vi "Read_DID.vi"() -> ()   [LabVIEW 2014]
uses:
  housekeeper/MSI/MSI typedefs/MSI.ctl
  <vilib>/Utility/error.llb/DialogType.ctl
panel:
  out "instant datarun":T1
  out "time stamp":timestamp
  in  "stop instantaneous loop":bool
  out "Shot collection loop":i32
  out "North discharge voltage":sgl[](graph)
  out "NDV error":errorcluster
  out "North discharge current":sgl[](graph)
  out "NDC error":errorcluster
  out "Shots in queue":i32
  out "Data request error":errorcluster
  in  "stop TCP listen":bool
  in  "Num diodes":i32=3
  in  "Num interferometers":i32=1
  out "Shot send loop":i32
  out "MSI+DID string length":i32
  out "TCP error":errorcluster
  out "Queue overflowed":bool
  in  "stop TCP":bool
  in  "stop DID":bool
  out "Data run status":T2 {"Timestamp" format="%#_8g"}
  out "MSI timed out":bool
  out "MSI error":errorcluster
  out "MSI":T3={"Timestamp"=0.0, "Discharge"={"Data valid"=FALSE, "Discharge current"=[], "Cathode anode voltage"=[], "Pulse length"=0.0, "Peak current"=0.0, "Bank voltage"=0.0}, "Heater"={"Data valid"=FALSE, "Heater current"=0.0, "Heater voltage"=0.0, "Heater temperature"=0.0}, "Gas pressure"={"Ion gauge data valid"=FALSE, "RGA data valid"=FALSE, "Fill pressure"=0.0, "Peak AMU"=0.0, "RGA partial pressures"=[]}, "Magnetic field"={"Data valid"=FALSE, "Magnetic field profile"=[], "Magnet power supply currents"=[], "Peak magnetic field"=0.0}, "Interferometer array"=[{"Data valid"=TRUE, "Interferometer"=[1200000000000.0, 1300000000000.0, 1500000000000.0, 1400000000000.0], "Peak density"=347.7}, {"Data valid"=TRUE, "Interferometer"=[1330000000000.0, 1450000000000.0, 1430000000000.0, 1560000000000.0], "Peak density"=654.9}, {"Data valid"=TRUE, "Interferometer"=[1110000000000.0, 1130000000000.0, 1440000000000.0, 1250000000000.0], "Peak density"=45.0}]} {"Timestamp" format="%<%X\n%x>T"}
  out "No discharge":bool
  in  "Write DID to file?":bool=TRUE
  out "File error":errorcluster
  out "Run error":errorcluster
  out "DID+MSI string":string
  out "Save path":path
  out "Data run timed out":bool
  out "Diode array":dbl[][](graph)
  out "Diode array":waveform(dbl)[](array[waveform])
  out "Diode error":errorcluster
  out "Micorwave array":dbl[][](graph)
  out "Microwave array":waveform(dbl)[](array[waveform])
  out "MArray error":errorcluster
  out "Discharge voltage":sgl[](graph)
  out "DV error":errorcluster
  out "Discharge current":sgl[](graph)
  out "DC error":errorcluster
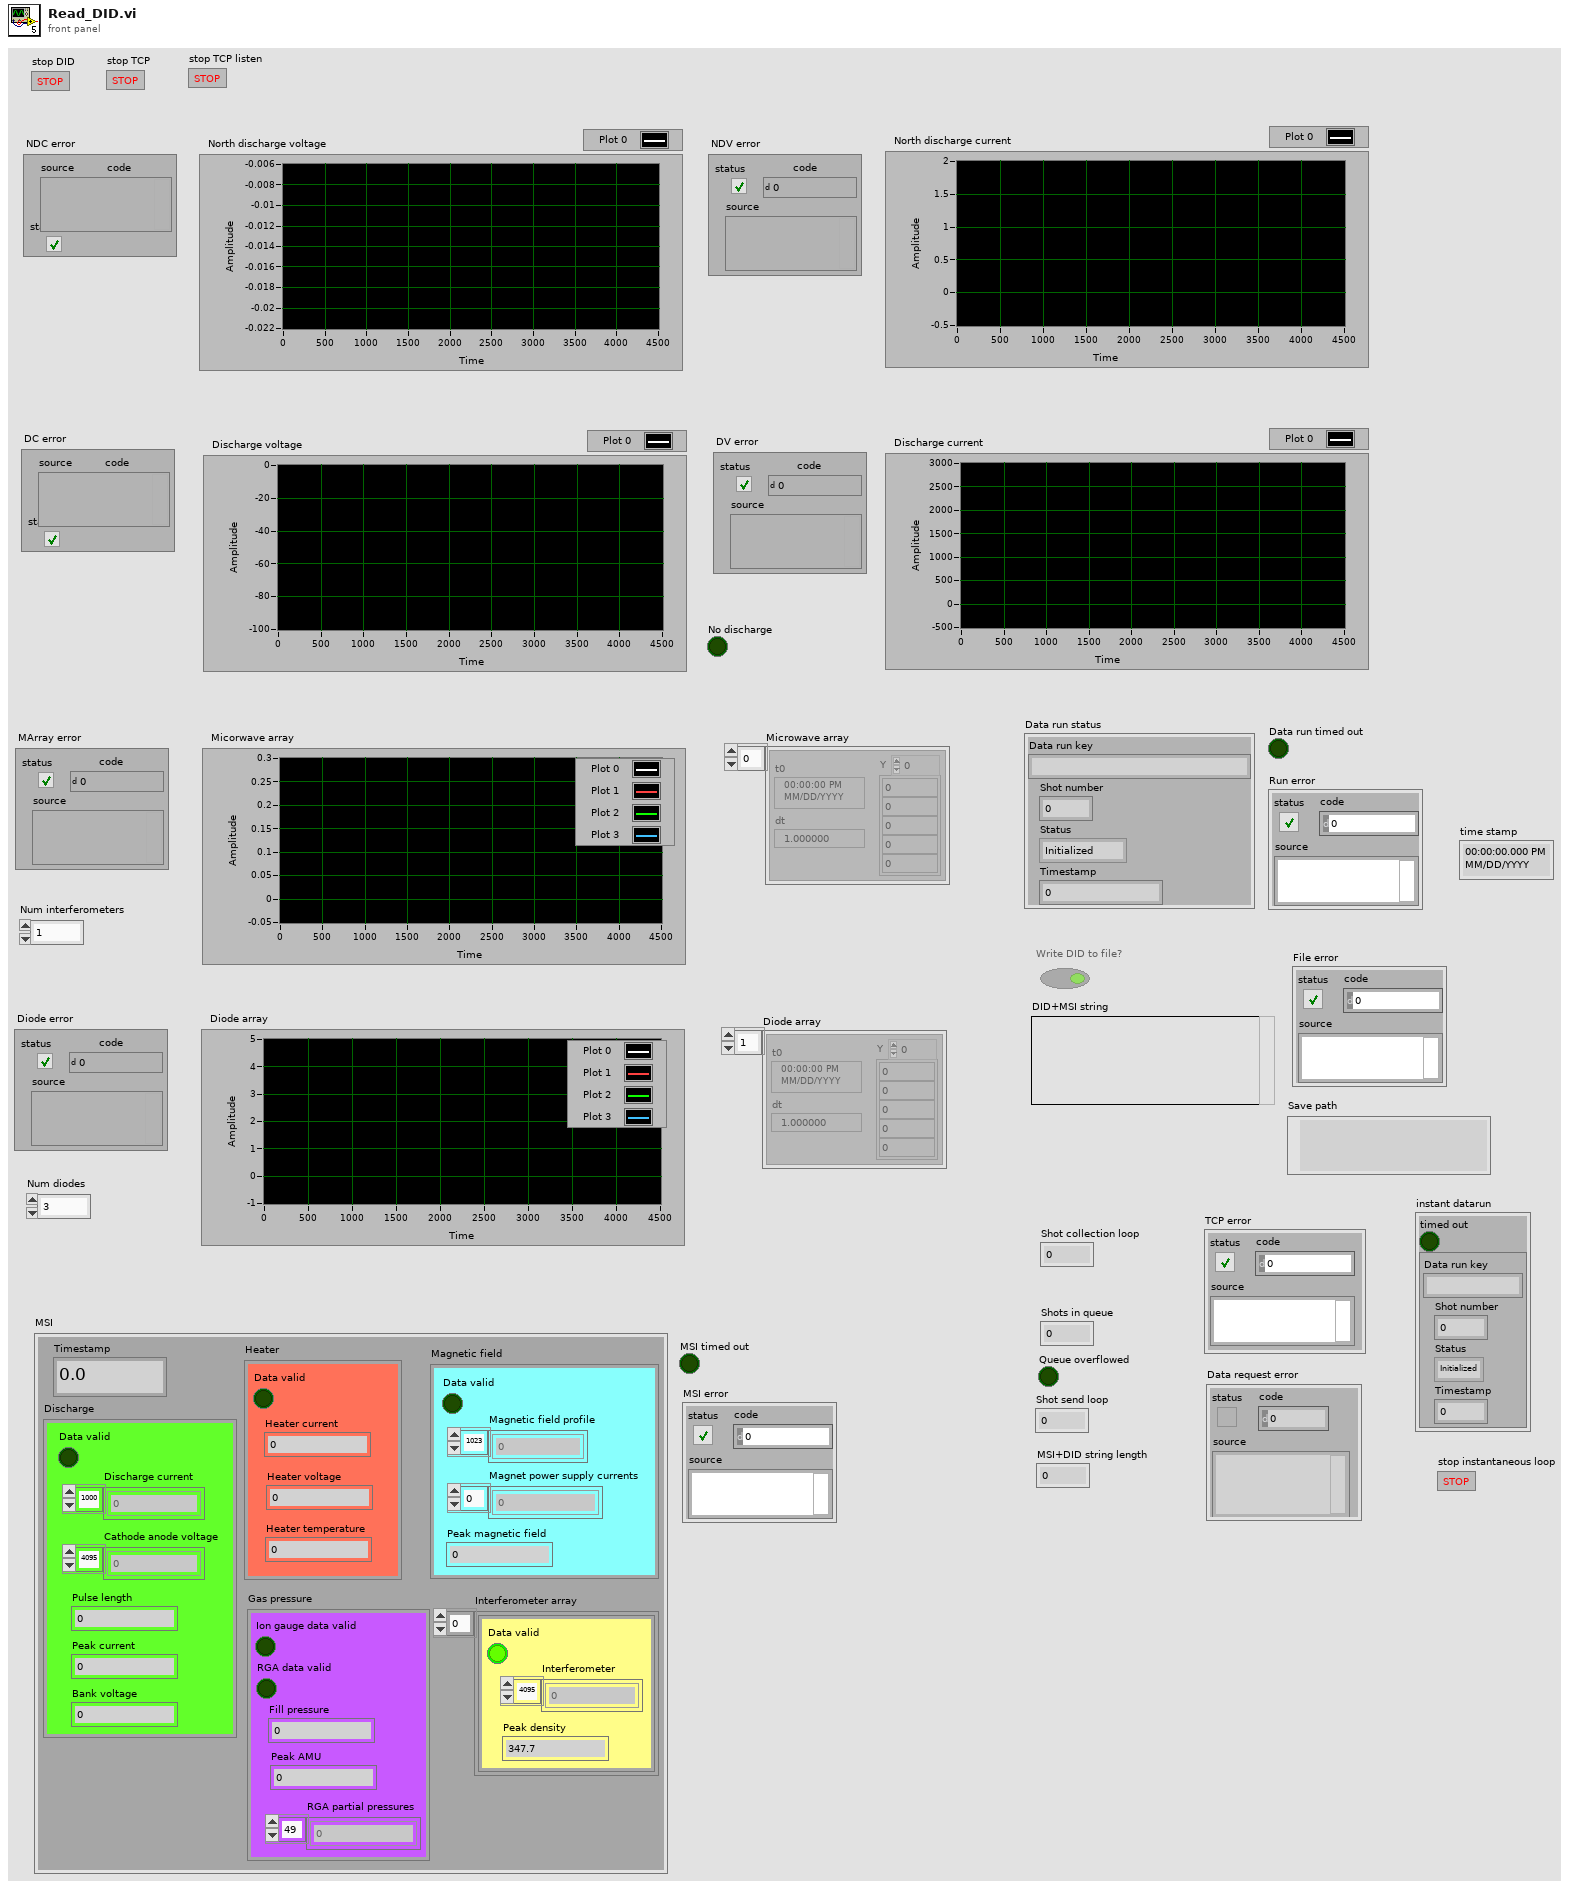
[diagram p1: front panel]
types:
  T1 = cluster{"timed out":bool, cluster{"Data run key":string, "Shot number":u32, "Status":enum16{"Initialized", "Running", "Aborted", "Default"}, "Timestamp":dbl}}
  T2 = cluster{"Data run key":string, "Shot number":u32, "Status":enum16{"Initialized", "Running", "Aborted", "Default"}, "Timestamp":dbl}
  T3 = typedef "MSI.ctl" = cluster{"Timestamp":dbl, "Discharge":cluster{"Data valid":bool, "Discharge current":sgl[], "Cathode anode voltage":sgl[], "Pulse length":sgl, "Peak current":sgl, "Bank voltage":sgl}, "Heater":cluster{"Data valid":bool, "Heater current":sgl, "Heater voltage":sgl, "Heater temperature":sgl}, "Gas pressure":cluster{"Ion gauge data valid":bool, "RGA data valid":bool, "Fill pressure":sgl, "Peak AMU":sgl, "RGA partial pressures":sgl[]}, "Magnetic field":cluster{"Data valid":bool, "Magnetic field profile":sgl[], "Magnet power supply currents":sgl[], "Peak magnetic field":sgl}, "Interferometer array":cluster{"Data valid":bool, "Interferometer":sgl[], "Peak density":sgl}[]}
  T4 = enum16{"Initialized", "Running", "Aborted", "Default"}
  T5 = enum16{"open", "replace", "create", "open or create", "replace or create", "replace or create with confirmation"}
  T6 = cluster{bool, cluster{"Data run key":string, "Shot number":u32, "Status":enum16{"Initialized", "Running", "Aborted", "Default"}, "Timestamp":dbl}}
  T7 = typedef "DialogType.ctl" = u16
  T8 = cluster{"Data valid":bool, "Heater current":sgl, "Heater voltage":sgl, "Heater temperature":sgl}
  T9 = cluster{"Ion gauge data valid":bool, "RGA data valid":bool, "Fill pressure":sgl, "Peak AMU":sgl, "RGA partial pressures":sgl[]}
  T10 = cluster{"Data valid":bool, "Magnetic field profile":sgl[], "Magnet power supply currents":sgl[], "Peak magnetic field":sgl}
  T11 = cluster{"timed out":bool, "Timestamp":dbl, "Heater":cluster{"Data valid":bool, "Heater current":sgl, "Heater voltage":sgl, "Heater temperature":sgl}, "Gas pressure":cluster{"Ion gauge data valid":bool, "RGA data valid":bool, "Fill pressure":sgl, "Peak AMU":sgl, "RGA partial pressures":sgl[]}, "Magnetic field":cluster{"Data valid":bool, "Magnetic field profile":sgl[], "Magnet power supply currents":sgl[], "Peak magnetic field":sgl}}
  T12 = cluster{"Waveform Graph 4":sgl[], "Waveform Graph 4":sgl[], "Waveform Graph 4":sgl[], "Waveform Graph 4":sgl[], "Y":dbl[][], timestamp[], dbl[], "Y":dbl[][], timestamp[], dbl[], "timed out":bool, cluster{"Data run key":string, "Shot number":u32, "Status":enum16{"Initialized", "Running", "Aborted", "Default"}, "Timestamp":dbl}}
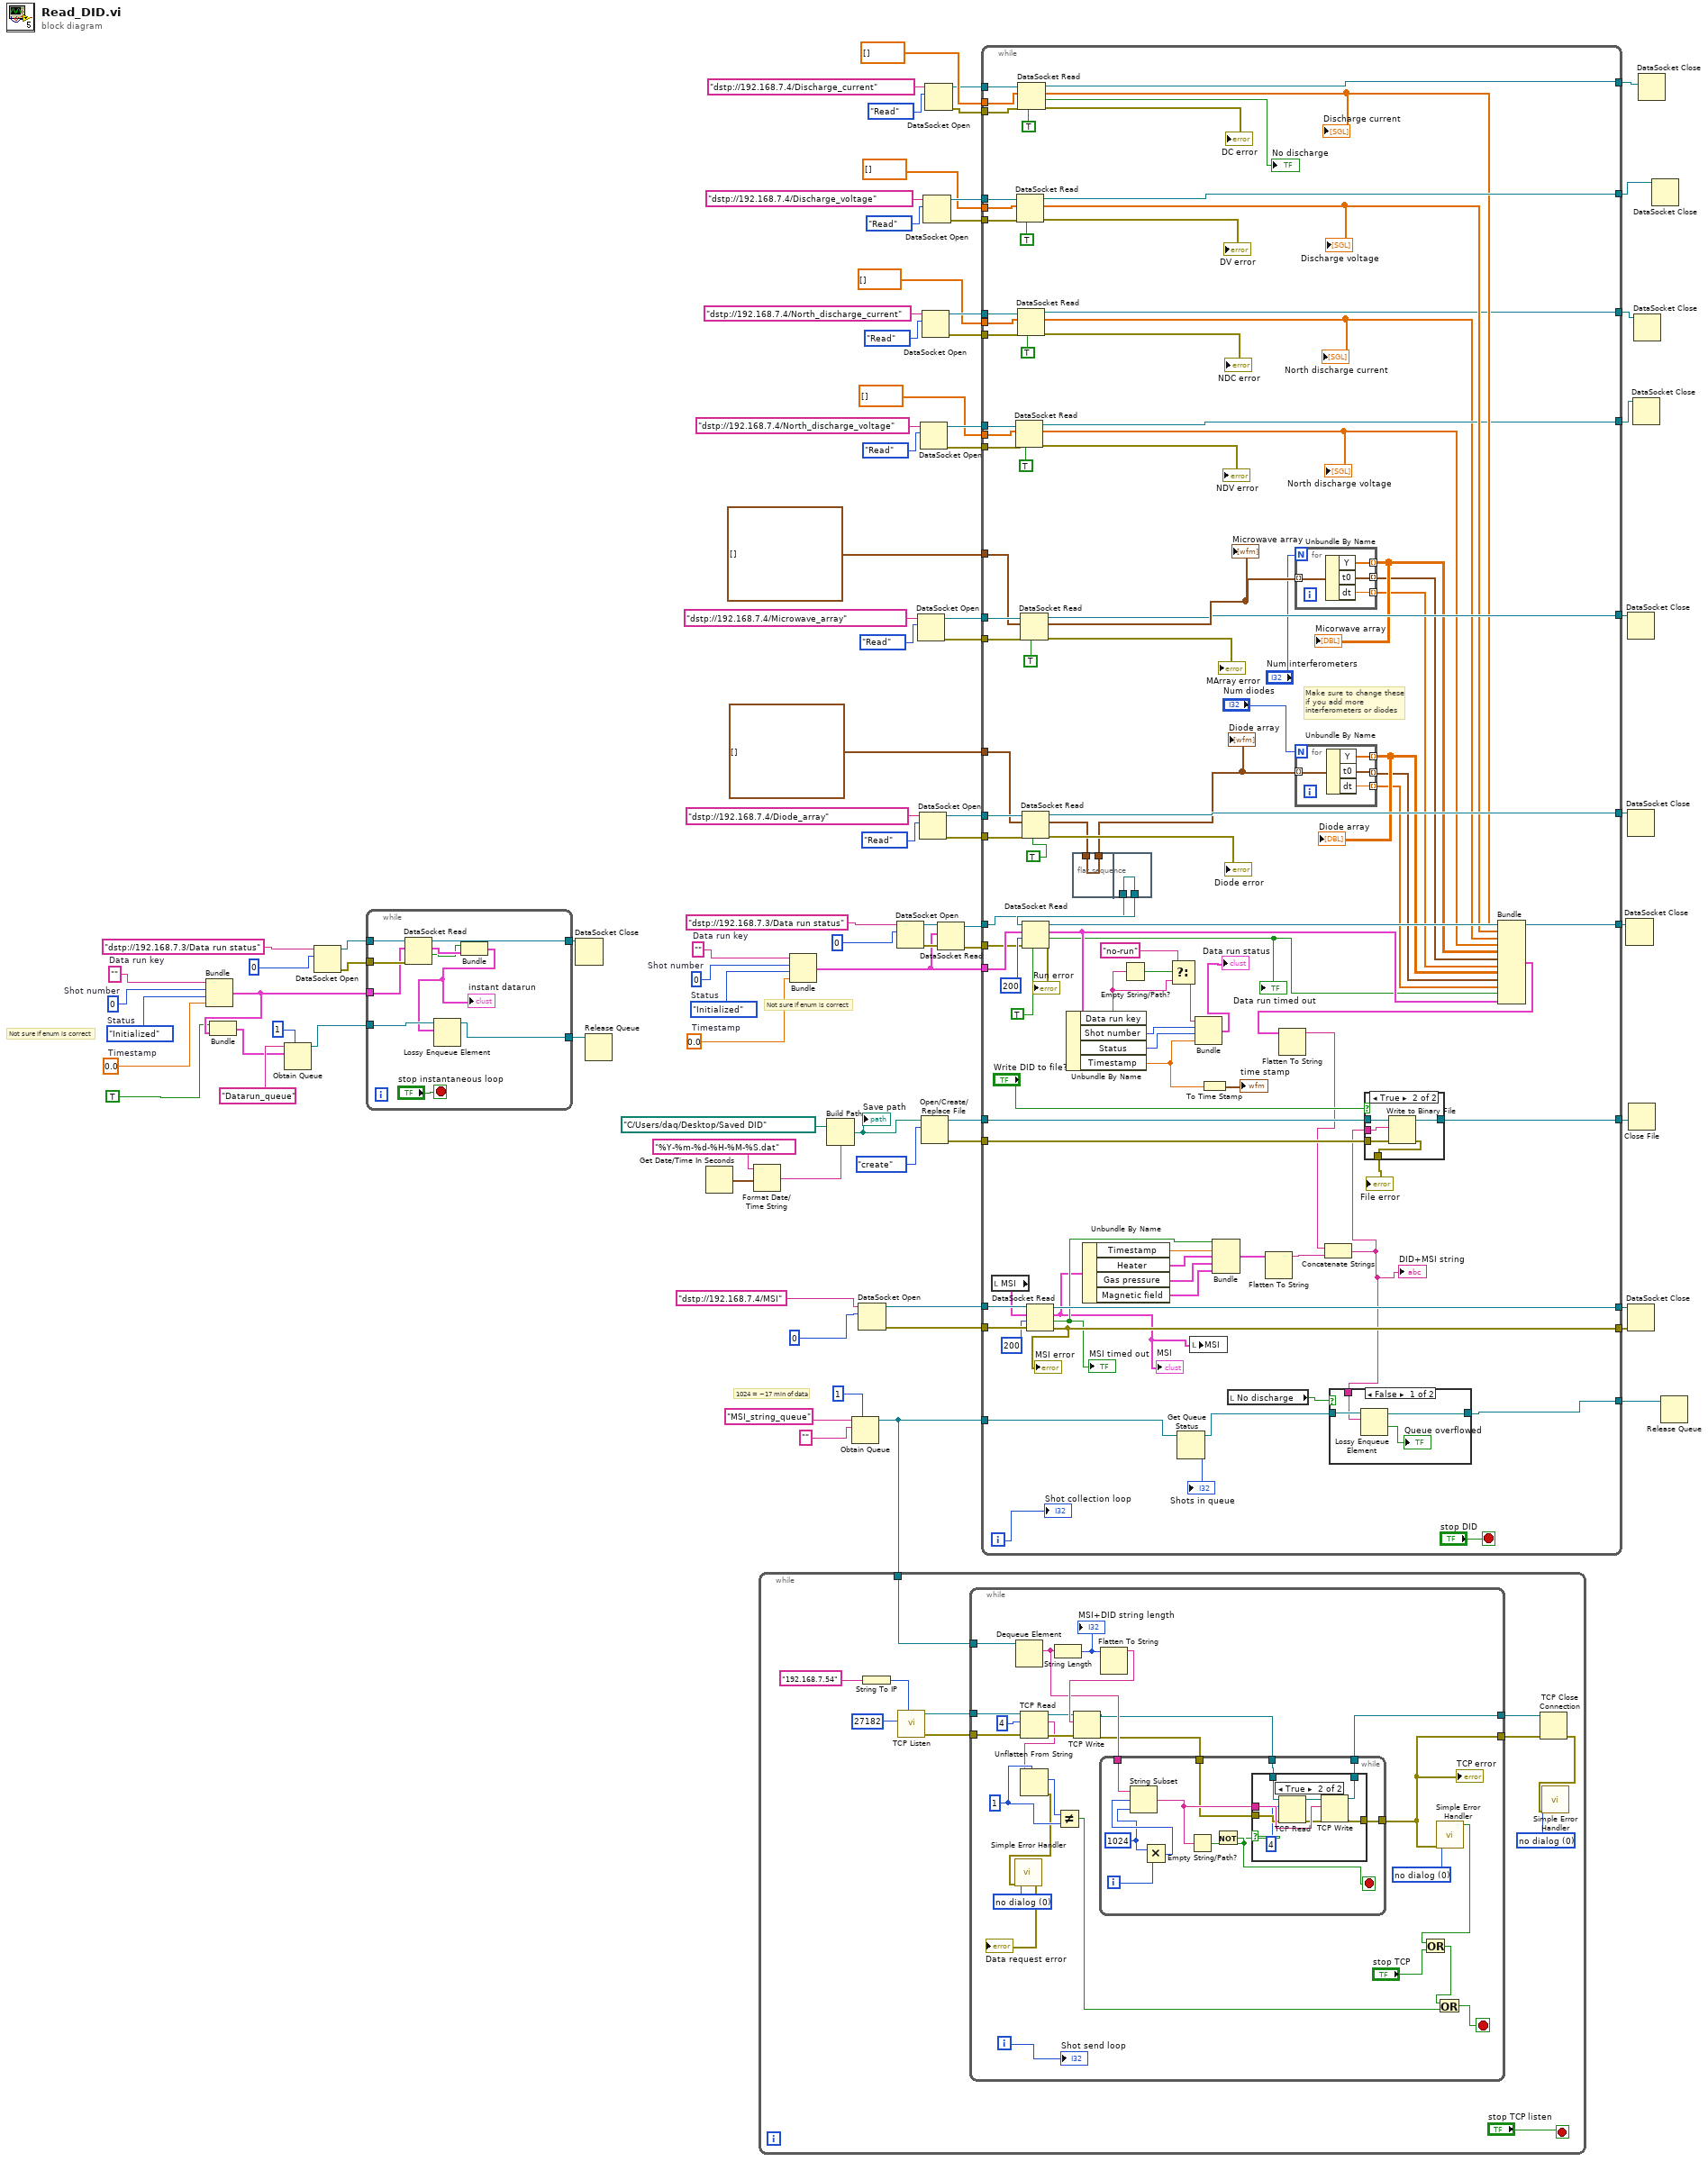
[diagram p0: block diagram]
diagram:
  w19 = 0.0  # Timestamp
  w18 = T4."Initialized"  # Status
  w17 = u32 0  # Shot number
  w16 = ""  # Data run key
  (unwired) sgl[] [] ("Waveform Graph 4")
  w63 = 0.0  # Timestamp
  w62 = T4."Initialized"  # Status
  w61 = u32 0  # Shot number
  w60 = ""  # Data run key
  (unwired) sgl[] [] ("Waveform Graph 4")
  # "Not sure if enum is correct"
  # "1024 = ~17 min of data"
  # "Not sure if enum is correct"
  n1 = Bundle("Data run key"=w16, "Shot number"=w17, "Status"=w18, "Timestamp"=w19) -> (w9:T2)  [unwired: 1 in]
  n2 = Bundle(TRUE, w9) -> (w7:T6)  [unwired: 1 in]
  n3 = Obtain Queue(max queue size (-1, unlimited)=1, name (unnamed)="Datarun_queue", element data type=w7) -> (queue out=w6:refnum<queue>)  [unwired: 2 in, 2 out]
  n4 = DataSocket Open(10:0, 11:"dstp://192.168.7.3/Data run status") -> (0:w13:errorcluster, 3:w15:refnum<k13>)  [unwired: 2 in]
  n5 = while {
    tunnel: w15 -> [w94]
    tunnel: [w93] -> w14
    tunnel: w13 -> [w92]
    tunnel: w9 -> [w91]
    tunnel: w6 -> [w89]
    tunnel: [w88] -> w10
    stop <- "stop instantaneous loop" stop-if-true
    n6 = DataSocket Read(8:w92, 10:w91, 11:w94) -> (1:w86:bool, 2:w87:T2, 3:w93:refnum<k13>)  [unwired: 2 in, 4 out]
    n7 = Bundle("timed out"=w86, w87) -> (w85:T1)  [unwired: 1 in]
    "instant datarun" <- w85
    n8 = Lossy Enqueue Element(queue=w89, element=w85) -> (queue out=w88:refnum<queue>)  [unwired: 1 in, 3 out]
  }
  n9 = DataSocket Close(11:w14) -> ()  [unwired: 2 in, 2 out]
  n10 = Release Queue(queue=w10) -> ()  [unwired: 2 in, 3 out]
  n11 = Get Date/Time In Seconds() -> (seconds since 1Jan1904=w57:timestamp)
  n12 = Format Date/Time String(time format string (%c)="%Y-%m-%d-%H-%M-%S.dat", seconds (now)=w57) -> (date/time string=w55:string)  [unwired: 1 in]
  n13 = Bundle("Data run key"=w60, "Shot number"=w61, "Status"=w62, "Timestamp"=w63) -> (w1:T2)  [unwired: 1 in]
  n14 = Build Path(base path=path "C:/Users/daq/Desktop/Saved DID", name or relative path=w55) -> (appended path=w53:path)
  "Save path" <- w53
  n15 = Obtain Queue(max queue size (-1, unlimited)=1, name (unnamed)="MSI_string_queue", element data type="" ("name (unnamed)")) -> (queue out=w36:refnum<queue>)  [unwired: 2 in, 2 out]
  n16 = while {
    tunnel: w36 -> [w98]
    stop <- "stop TCP listen" stop-if-true
    w95 = T7 0 items=["no dialog", "OK message", "continue or stop message", "OK message + warnings", "continue/stop + warnings"] ("type of dialog (OK msg:1)")
    n17 = String To IP(1:"192.168.7.54" ("name (unnamed)")) -> (0:w99:u32)
    n18 = call <vilib>:"TCP Listen.vi"("net address"=w99, "port"=u16 27182) -> ("error out"=w105:errorcluster, "connection ID"=w101:refnum<k5>)  [unwired: 5 in, 3 out]
    n19 = while {
      tunnel: w98 -> [w131]
      tunnel: w101 -> [w119]
      tunnel: [w127] -> w102
      tunnel: [w122] -> w103
      tunnel: w105 -> [w118]
      i -> [w126]
      stop <- w111 stop-if-true
      w107 = T7 0 items=["no dialog", "OK message", "continue or stop message", "OK message + warnings", "continue/stop + warnings"] ("type of dialog (OK msg:1)")
      w115 = 1
      w121 = T7 0 items=["no dialog", "OK message", "continue or stop message", "OK message + warnings", "continue/stop + warnings"] ("type of dialog (OK msg:1)")
      n20 = Dequeue Element(queue=w131) -> (element=w128:string)  [unwired: 2 in, 3 out]
      n21 = TCP Read(connection ID=w119, bytes to read=4, error in (no error)=w118) -> (connection ID out=w117:refnum<k5>, data out=w109:string, error out=w116:errorcluster)  [unwired: 2 in]
      n22 = Unflatten From String(type=w115, binary string=w109) -> (value=w114:i32, error out=w108:errorcluster)  [unwired: 3 in, 1 out]
      n23 = call <vilib>:"Simple Error Handler.vi"("type of dialog (OK msg:1)"=w107, "error in (no error)"=w108) -> ("error out"=→"Data request error":errorcluster)  [unwired: 3 in, 4 out]
      n24 = String Length(string=w128) -> (length=w130:i32)
      "MSI+DID string length" <- w130
      n25 = Not Equal?(x=w114, y=w115) -> (x != y?=w113:bool)
      n26 = Flatten To String(anything=w130) -> (data string=w129:string)  [unwired: 3 in, 2 out]
      n27 = TCP Write(connection ID=w117, data in=w129, error in (no error)=w116) -> (connection ID out=w125:refnum<k5>, error out=w124:errorcluster)  [unwired: 1 in, 1 out]
      n28 = while {
        tunnel: w128 -> [w142]
        tunnel: w125 -> [w136]
        tunnel: w124 -> [w135]
        tunnel: [w134] -> w127
        tunnel: [w133] -> w122
        i -> [w141]
        stop <- w139 stop-if-true
        w132 = 1024 ("x")
        n29 = Multiply(x=w132, y=w141) -> (x*y=w140:i32)
        n30 = String Subset(string=w142, offset (0)=w140, length (rest)=w132) -> (substring=w137:string)
        n31 = Empty String/Path?(string/path=w137) -> (empty?=w139:bool)
        n32 = Not(x=w139) -> (.not. x?=w138:bool)
        n33 = case shown="True" w138 {
          tunnel: w137 -> [_ w148]
          tunnel: w136 -> [w143 w150]
          tunnel: w135 -> [w144 w147]
          tunnel: [w143 w152] -> w134
          tunnel: [w144 w151] -> w133
          frame False {
          }
          frame True {
            n34 = TCP Read(connection ID=w150, bytes to read=4, error in (no error)=w147) -> (connection ID out=w149:refnum<k5>, error out=w146:errorcluster)  [unwired: 2 in, 1 out]
            n35 = TCP Write(connection ID=w149, data in=w148, error in (no error)=w146) -> (connection ID out=w152:refnum<k5>, error out=w151:errorcluster)  [unwired: 1 in, 1 out]
          }
        }
      }
      "TCP error" <- w122
      n36 = call <vilib>:"Simple Error Handler.vi"("type of dialog (OK msg:1)"=w121, "error in (no error)"=w122) -> ("error?"=w120:bool)  [unwired: 3 in, 4 out]
      n37 = Or(x=w120, y="stop TCP") -> (x .or. y?=w112:bool)
      n38 = Or(x=w112, y=w113) -> (x .or. y?=w111:bool)
      "Shot send loop" <- w126
    }
    n39 = TCP Close Connection(connection ID=w102, error in (no error)=w103) -> (error out=w96:errorcluster)  [unwired: 1 in, 1 out]
    n40 = call <vilib>:"Simple Error Handler.vi"("type of dialog (OK msg:1)"=w95, "error in (no error)"=w96) -> ()  [unwired: 3 in, 5 out]
  }
  n41 = DataSocket Open(10:0, 11:"dstp://192.168.7.4/MSI") -> (0:w43:errorcluster, 3:w44:refnum<k13>)  [unwired: 2 in]
  n42 = DataSocket Open(10:0, 11:"dstp://192.168.7.3/Data run status") -> (0:w3:errorcluster, 3:w5:refnum<k13>)  [unwired: 2 in]
  n43 = DataSocket Open(10:enum16{"Read"}."Read", 11:"dstp://192.168.7.4/Microwave_array" ("String")) -> (0:w49:errorcluster, 3:w73:refnum<k13>)  [unwired: 2 in]
  n44 = DataSocket Open(10:enum16{"Read"}."Read", 11:"dstp://192.168.7.4/Diode_array" ("String")) -> (0:w48:errorcluster, 3:w72:refnum<k13>)  [unwired: 2 in]
  n45 = DataSocket Open(10:enum16{"Read"}."Read", 11:"dstp://192.168.7.4/North_discharge_voltage" ("String")) -> (0:w22:errorcluster, 3:w24:refnum<k13>)  [unwired: 2 in]
  n46 = Open/Create/Replace File(file path (use dialog)=w53, operation (0:open)=T5."create" ("operation")) -> (refnum out=w52:refnum<file>, error out=w51:errorcluster)  [unwired: 4 in, 1 out]
  n47 = DataSocket Open(10:enum16{"Read"}."Read", 11:"dstp://192.168.7.4/North_discharge_current" ("String")) -> (0:w28:errorcluster, 3:w29:refnum<k13>)  [unwired: 2 in]
  n48 = DataSocket Open(10:enum16{"Read"}."Read", 11:"dstp://192.168.7.4/Discharge_voltage" ("String")) -> (0:w50:errorcluster, 3:w74:refnum<k13>)  [unwired: 2 in]
  n49 = DataSocket Open(10:enum16{"Read"}."Read", 11:"dstp://192.168.7.4/Discharge_current" ("String")) -> (0:w35:errorcluster, 3:w75:refnum<k13>)  [unwired: 2 in]
  n50 = DataSocket Read(8:w3, 10:w1, 11:w5) -> (0:w2:errorcluster, 3:w4:refnum<k13>)  [unwired: 2 in, 5 out]
  n51 = while {
    tunnel: sgl[] [] ("Waveform Graph 4") -> [w243]
    tunnel: w75 -> [w242]
    tunnel: w74 -> [w241]
    tunnel: w73 -> [w240]
    tunnel: w72 -> [w239]
    tunnel: waveform(dbl)[] [] -> [w238]
    tunnel: waveform(dbl)[] [] -> [w237]
    tunnel: sgl[] [] ("Waveform Graph 4") -> [w236]
    tunnel: [w235] -> w30
    tunnel: [w234] -> w68
    tunnel: [w233] -> w67
    tunnel: [w232] -> w66
    tunnel: w4 -> [w155]
    tunnel: w1 -> [w230]
    tunnel: [w229] -> w59
    tunnel: w52 -> [w214]
    tunnel: w51 -> [w213]
    tunnel: w50 -> [w228]
    tunnel: w49 -> [w227]
    tunnel: w48 -> [w226]
    tunnel: w2 -> [w225]
    tunnel: [w196] -> w47
    tunnel: w44 -> [w211]
    tunnel: w43 -> [w210]
    tunnel: [w208] -> w42
    tunnel: [w207] -> w41
    tunnel: w36 -> [w192]
    tunnel: [w160] -> w37
    tunnel: w35 -> [w183]
    tunnel: w29 -> [w173]
    tunnel: w28 -> [w172]
    tunnel: sgl[] [] ("Waveform Graph 4") -> [w171]
    tunnel: [w170] -> w26
    tunnel: [w169] -> w25
    tunnel: w24 -> [w168]
    tunnel: sgl[] [] ("Waveform Graph 4") -> [w167]
    tunnel: w22 -> [w166]
    i -> [w163]
    stop <- "stop DID" stop-if-true
    # "Make sure to change these if you add more interferometers or diodes"
    n52 = local read "MSI"() -> (w197:T3)
    n53 = DataSocket Read(6:TRUE ("wait for updated value (T)"), 8:w166, 10:w167, 11:w168) -> (0:→"NDV error":errorcluster, 2:w164:sgl[], 3:w169:refnum<k13>)  [unwired: 1 in, 4 out]
    "North discharge voltage" <- w164
    n54 = DataSocket Read(6:TRUE ("wait for updated value (T)"), 8:w228, 10:w236, 11:w241) -> (0:→"DV error":errorcluster, 2:w178:sgl[], 3:w234:refnum<k13>)  [unwired: 1 in, 4 out]
    "Discharge voltage" <- w178
    n55 = DataSocket Read(6:TRUE ("wait for updated value (T)"), 8:w172, 10:w171, 11:w173) -> (0:→"NDC error":errorcluster, 2:w165:sgl[], 3:w170:refnum<k13>)  [unwired: 1 in, 4 out]
    "North discharge current" <- w165
    n56 = DataSocket Read(6:TRUE ("wait for updated value (T)"), 8:w183, 10:w243, 11:w242) -> (0:→"DC error":errorcluster, 1:→"No discharge":bool, 2:w179:sgl[], 3:w235:refnum<k13>)  [unwired: 1 in, 3 out]
    "Discharge current" <- w179
    n57 = DataSocket Read(6:TRUE ("wait for updated value (T)"), 8:w227, 10:w237, 11:w240) -> (0:→"MArray error":errorcluster, 2:w247:waveform(dbl)[], 3:w233:refnum<k13>)  [unwired: 1 in, 4 out]
    "Microwave array" <- w247
    n58 = DataSocket Read(6:TRUE ("wait for updated value (T)"), 8:w226, 10:w238, 11:w239) -> (0:→"Diode error":errorcluster, 2:w153:waveform(dbl)[], 3:w232:refnum<k13>)  [unwired: 1 in, 4 out]
    n59 = DataSocket Read(6:TRUE ("wait for updated value (T)"), 8:w225, 9:200, 10:w230, 11:w156) -> (0:→"Run error":errorcluster, 1:w158:bool, 2:w159:T2, 3:w229:refnum<k13>)  [unwired: 3 out]
    "Data run timed out" <- w158
    n60 = DataSocket Read(8:w210, 9:200 ("ms timeout (10000)"), 10:w197, 11:w211) -> (0:w207:errorcluster, 1:w199:bool, 2:w198:T3, 3:w208:refnum<k13>)  [unwired: 1 in, 3 out]
    "MSI" <- w198
    "MSI error" <- w207
    "MSI timed out" <- w199
    n61 = Unbundle By Name(w159) -> ("Data run key"=w188:string, "Shot number"=w186:u32, "Status"=w185:T4, "Timestamp"=w162:dbl)
    n62 = flat-sequence {
      tunnel: [w253] -> w154
      tunnel: w153 -> [w253]
      tunnel: [w254] -> w156
      tunnel: w155 -> [w254]
      frame #0 {
      }
      frame #1 {
      }
    }
    n63 = Unbundle By Name(w198) -> ("Timestamp"=w206:dbl, "Heater"=w205:T8, "Gas pressure"=w204:T9, "Magnetic field"=w203:T10)
    n64 = Empty String/Path?(string/path=w188) -> (empty?=w190:bool)
    n65 = Select(t="no-run", s=w190, f=w188) -> (s? t:f=w187:string)
    n66 = Get Queue Status(queue=w192) -> (queue out=w182:refnum<queue>, # elements in queue=→"Shots in queue":i32)  [unwired: 2 in, 6 out]
    n67 = local write "MSI"(w198) -> ()
    n68 = Bundle("Data run key"=w187, "Shot number"=w186, "Status"=w185, "Timestamp"=w162) -> (→"Data run status":T2)  [unwired: 1 in]
    n69 = To Time Stamp(1:w162) -> (0:→"time stamp":timestamp)
    n70 = Bundle("timed out"=w199, "Timestamp"=w206, "Heater"=w205, "Gas pressure"=w204, "Magnetic field"=w203) -> (w202:T11)  [unwired: 1 in]
    n71 = local read "No discharge"() -> (w180:bool)
    n72 = Flatten To String(anything=w202) -> (data string=w200:string)  [unwired: 3 in, 2 out]
    n73 = for {
      N: "Num interferometers" -> [_]
      tunnel: w247 -> [w274] mode=indexing
      tunnel: [w273] -> w221 mode=indexing
      tunnel: [w272] -> w222 mode=indexing
      tunnel: [w271] -> w220 mode=indexing
      n74 = Unbundle By Name(w274) -> ("Y"=w272:dbl[], "t0"=w273:timestamp, "dt"=w271:dbl)
    }
    "Micorwave array" <- w222
    n75 = for {
      N: "Num diodes" -> [_]
      tunnel: w154 -> [w270] mode=indexing
      tunnel: [w269] -> w219 mode=indexing
      tunnel: [w268] -> w218 mode=indexing
      tunnel: [w267] -> w217 mode=indexing
      n76 = Unbundle By Name(w270) -> ("Y"=w269:dbl[], "t0"=w268:timestamp, "dt"=w267:dbl)
    }
    "Diode array" <- w219
    n77 = Bundle("Waveform Graph 4"=w179, "Waveform Graph 4"=w178, "Waveform Graph 4"=w165, "Waveform Graph 4"=w164, "Y"=w222, w221, w220, "Y"=w219, w218, w217, "timed out"=w158, w159) -> (w223:T12)  [unwired: 1 in]
    n78 = Flatten To String(anything=w223) -> (data string=w201:string)  [unwired: 3 in, 2 out]
    n79 = Concatenate Strings(w201, w200) -> (w181:string)
    "DID+MSI string" <- w181
    n80 = case shown="False" w180 {
      tunnel: w182 -> [w257 w259]
      tunnel: [w256 w259] -> w160
      tunnel: w181 -> [w255 _]
      frame False {
        n81 = Lossy Enqueue Element(queue=w257, element=w255) -> (queue out=w256:refnum<queue>, overflow?=→"Queue overflowed":bool)  [unwired: 1 in, 2 out]
      }
      frame True {
      }
    }
    n82 = case shown="True" "Write DID to file?" {
      tunnel: [w260 w263] -> w215
      tunnel: w214 -> [w261 w266]
      tunnel: w213 -> [w260 w265]
      tunnel: [w261 w264] -> w196
      tunnel: w181 -> [_ w262]
      frame False {
      }
      frame True {
        n83 = Write to Binary File(file (use dialog)=w266, data=w262, error in=w265) -> (refnum out=w264:refnum<file>, error out=w263:errorcluster)  [unwired: 3 in, 1 out]
      }
    }
    "File error" <- w215
    "Diode array" <- w154
    "Shot collection loop" <- w163
  }
  n84 = DataSocket Close(11:w59) -> ()  [unwired: 2 in, 2 out]
  n85 = DataSocket Close(11:w67) -> ()  [unwired: 2 in, 2 out]
  n86 = DataSocket Close(11:w66) -> ()  [unwired: 2 in, 2 out]
  n87 = DataSocket Close(8:w41, 11:w42) -> ()  [unwired: 1 in, 2 out]
  n88 = Close File(refnum=w47) -> ()  [unwired: 1 in, 2 out]
  n89 = DataSocket Close(11:w25) -> ()  [unwired: 2 in, 2 out]
  n90 = DataSocket Close(11:w26) -> ()  [unwired: 2 in, 2 out]
  n91 = DataSocket Close(11:w30) -> ()  [unwired: 2 in, 2 out]
  n92 = DataSocket Close(11:w68) -> ()  [unwired: 2 in, 2 out]
  n93 = Release Queue(queue=w37) -> ()  [unwired: 2 in, 3 out]
